vi "Press Compensation.vi"(3 "P abs (mb)":dbl, 4 "Temperature (C)":dbl, 5 "Altitude (ft)":dbl=980.0) -> (0 "Pr Correction":dbl, 1 "Press_Hg":dbl format="%.2g", 2 "Press_hPa":dbl)   [LabVIEW 2014]
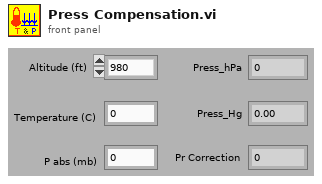
[diagram p1: front panel]
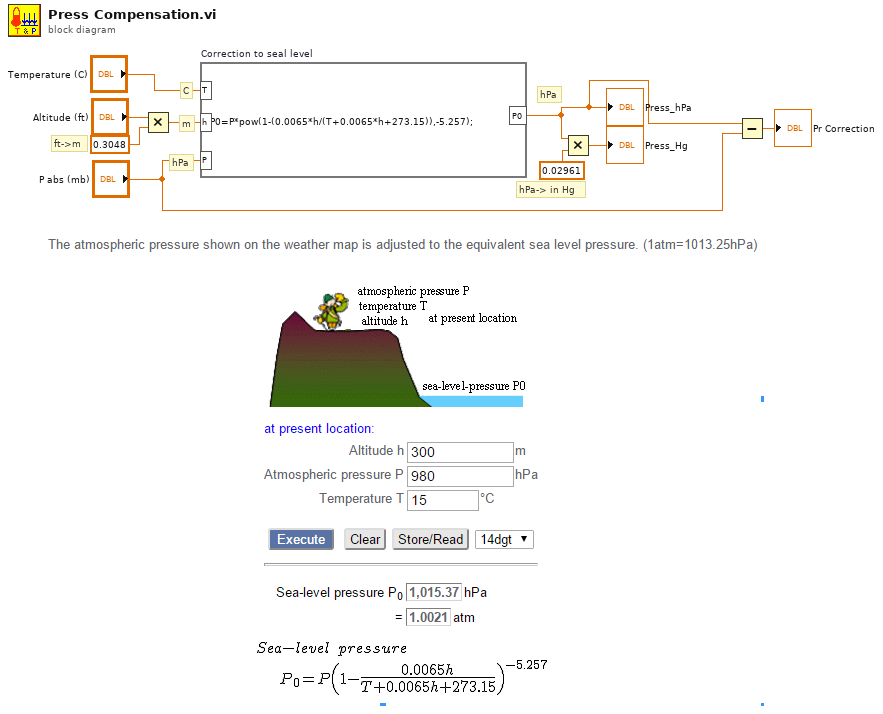
[diagram p0: block diagram]
diagram:
  # "ft->m"
  # "hPa-> in Hg"
  # "hPa"
  # "hPa"
  # "C"
  # "m"
  n1 = Multiply(x="Altitude (ft)", y=0.3048) -> (x*y=w7:dbl)
  n2 = formula code="P0=P*pow(1-(0.0065*h/(T+0.0065*h+273.15)),-5.257);" "Correction to seal level"("P"="P abs (mb)", "T"="Temperature (C)", "h"=w7) -> ("P0"=w3:dbl)
  "Press_hPa" <- w3
  n3 = Multiply(x=w3, y=0.02961) -> (x*y=→"Press_Hg":dbl)
  n4 = Subtract(x=w3, y="P abs (mb)") -> (x-y=→"Pr Correction":dbl)
